vi "LIDAR Compute Heading Angle (SubVI).vi"(10 "Y Array":dbl[](array[numeric]), 11 "X Array":dbl[](array[numeric])) -> (1 "LIDAR Computed Angle":dbl, 2 "intercept":dbl, 3 "slope":dbl)   [LabVIEW 2017]
uses:
  <vilib>/Analysis/NI_AALPro.lvlib
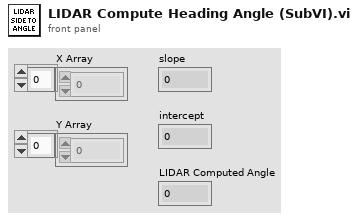
[diagram p1: front panel]
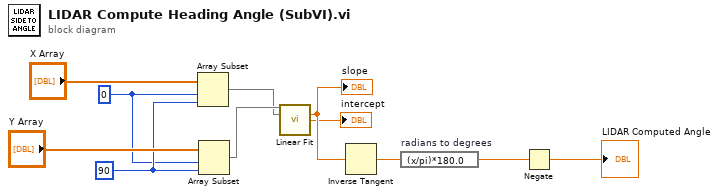
[diagram p0: block diagram]
diagram:
  w7 = 90 ("length")
  w6 = 0 ("index")
  n1 = Array Subset(array="X Array", index=w6, length=w7) -> (w10:dbl[])
  n2 = Array Subset(array="Y Array", index=w6, length=w7) -> (w11:dbl[])
  n3 = call <vilib>:"Linear Fit.vi"("Y"=w11, "X"=w10) -> ("slope"=w2:dbl, "intercept"=→"intercept":dbl)  [unwired: 9 in, 3 out]
  "slope" <- w2
  n4 = Inverse Tangent(1:w2) -> (0:w3:dbl)
  n5 = expression code="(x/pi)*180.0" "radians to degrees"(w3) -> (w4:dbl)
  n6 = Negate(x=w4) -> (-x=→"LIDAR Computed Angle":dbl)
